vi "freq file -- file select controller.vi"(6 "Sweep folder path":path=path "\\\\rus-one\\newdata/data/Ultrasound/Experiment/ProbeTest/Probe10/Hg1201-4-C199-80K-1/Sweep1", 7 "action":T3=enum."init", 8 "Numeric":dbl, 11 "file select ref":refnum<vi>) -> (0 "file select OUT":T1={"from file "="1827_a", "load"=FALSE, "read from file list"=0, "folder kind"=enum."9w"} {"read from file list" items=["769_a", "841_a", "1399_a", "1502_a", "1527_a", "1705_a", "1916_a", "1958_a", "2061_a", "2227_a", "2365_a", "2551_a", "2713_a", "2761_a", "2964_a", "3000_a", "3030_a", "3084_a", "3235_a", "3366_a"]}, 1 "Numeric out":dbl, 3 "file select ref out":refnum<vi>)   [LabVIEW 2015]
uses:
  save-read action.ctl
  freq file -- file select control.ctl
  freq file -- file select folder control.ctl
  D:/github/resonant_ultrasound/maglab ultrasound -- arkady/file -- 9w path.vi
  D:/github/resonant_ultrasound/maglab ultrasound -- arkady/file -- open-create folder.vi
  <vilib>/regexp/Match Regular Expression.xnode
panel:
  in  "folder kind":T2=enum."9w"
  in  "file select":T1={"from file "="1827_a", "load"=FALSE, "read from file list"=0, "folder kind"=enum."9w"} {"read from file list" items=["769_a", "841_a", "1399_a", "1502_a", "1527_a", "1705_a", "1916_a", "1958_a", "2061_a", "2227_a", "2365_a", "2551_a", "2713_a", "2761_a", "2964_a", "3000_a", "3030_a", "3084_a", "3235_a", "3366_a"]}
  in  "load":bool caption="read"
  in  "regexp":string="(from file).*"
  in  "read from file list":u16(ring) items=["769_a", "841_a", "1399_a", "1502_a", "1527_a", "1705_a", "1916_a", "1958_a", "2061_a", "2227_a", "2365_a", "2551_a", "2713_a", "2761_a", "2964_a", "3000_a", "3030_a", "3084_a", "3235_a", "3366_a"]
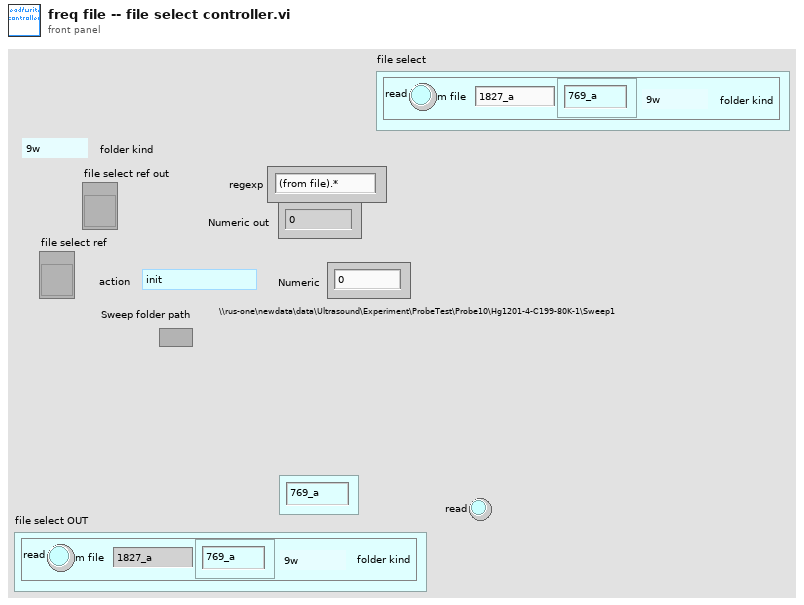
[diagram p1: front panel]
types:
  T1 = typedef "freq file -- file select control.ctl" = cluster{"from file ":string, "load":bool, "read from file list":u16, "folder kind":T2}
  T2 = typedef "freq file -- file select folder control.ctl" = enum16{"monitor", "9w"}
  T3 = typedef "save-read action.ctl" = enum16{"update save list", "update read list", "init", "check", "lookup read number", "lookup write number", "copy read from read ring", "saved file dirty", "saved file clean", "read file OK", "read file not OK", "nearest right", "nearest left", "increment read from", "copy read to save", "init save file", "erase event", "save event", "read event", "set save file", "decrement read from"}
  T4 = typedef "slide control.ctl" = cluster{"in slide":bool, "direction":bool, "start ":bool, "stop":bool, "next":bool}
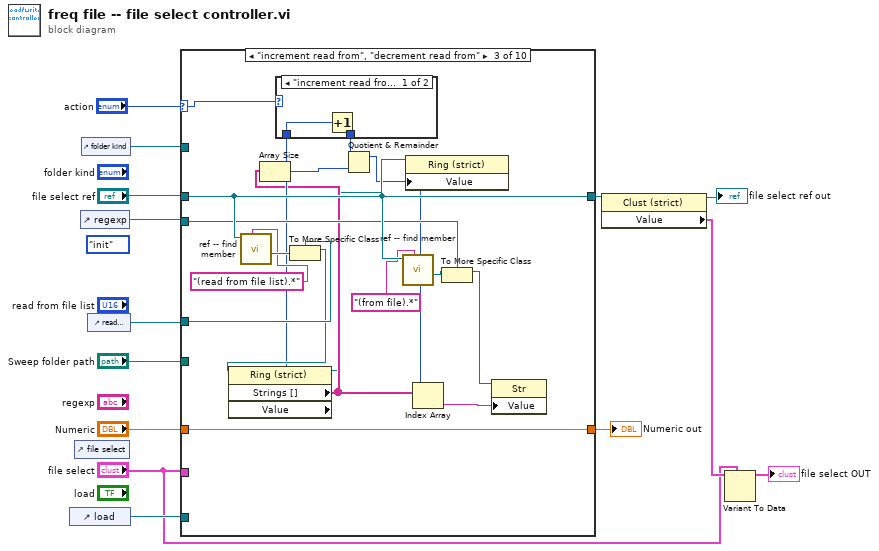
[diagram p0: block diagram]
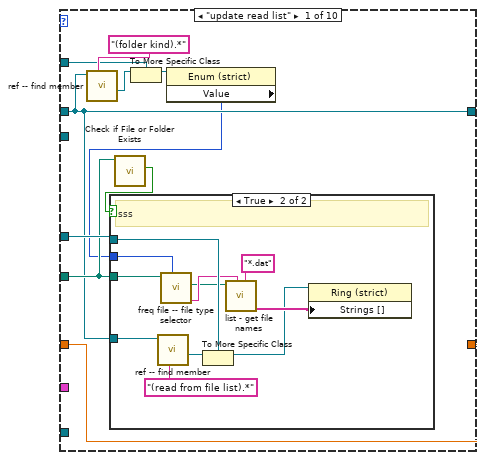
[diagram p2: hidden frame]
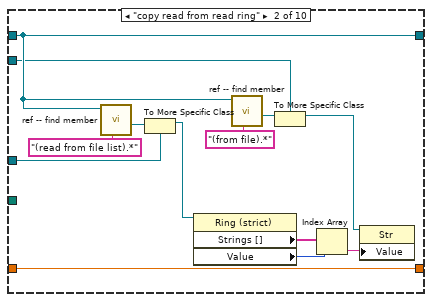
[diagram p4: hidden frame]
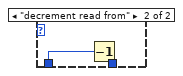
[diagram p5: hidden frame]
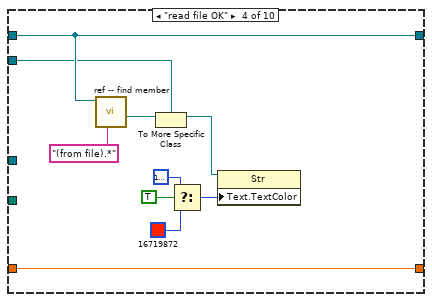
[diagram p6: hidden frame]
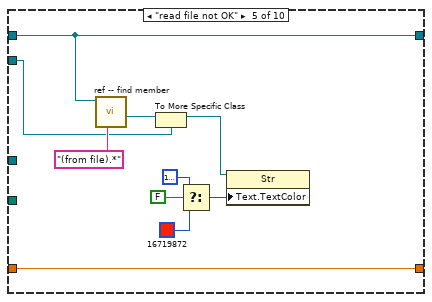
[diagram p7: hidden frame]
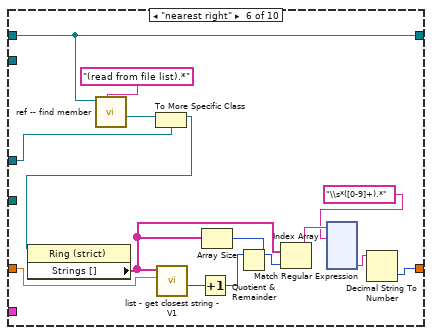
[diagram p8: hidden frame]
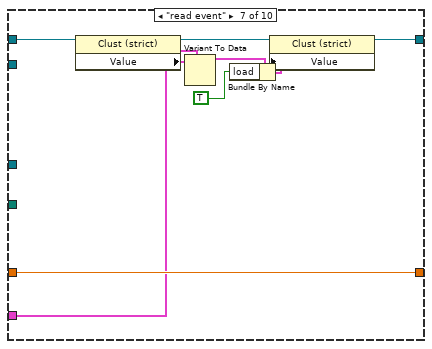
[diagram p9: hidden frame]
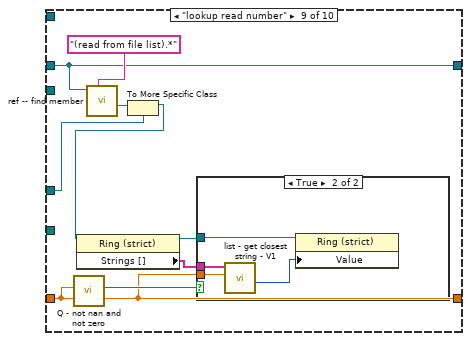
[diagram p11: hidden frame]
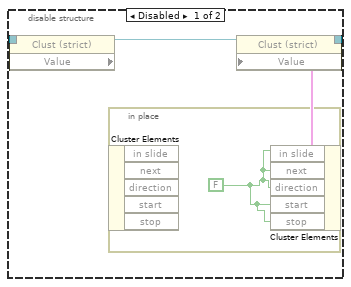
[diagram p14: hidden frame]
diagram:
  (unwired) save-read_action."init" ("action")
  n1 = control-ref of="load"() -> (w7:refnum<vi>)
  n2 = control-ref of="file select"() -> ()  [unwired: 1 out]
  n3 = control-ref of="regexp"() -> (w9:refnum<vi>)
  n4 = control-ref of="folder kind"() -> (w6:refnum<vi>)
  n5 = control-ref of="read from file list"() -> (w12:refnum<vi>)
  n6 = case shown="\"increment read from\", \"decrement read from\"" "action" {
    selector: "action" -> [_ _ w49 _ _ _ _ _ _ _]
    tunnel: "file select ref" -> [w19 w41 w61 w80 w90 w105 w225 w229 w232 w245]
    tunnel: [w19 w41 w61 w80 w90 w105 w222 w229 w232 w244] -> w2
    tunnel: "file select" -> [_ _ _ _ _ _ w224 _ _ _]
    tunnel: w12 -> [w24 w43 w63 _ _ w92 _ _ w235 _]
    tunnel: "Sweep folder path" -> [w23 _ _ _ _ _ _ _ _ _]
    tunnel: "Numeric" -> [w21 w36 w56 w71 w81 w91 w227 w228 w230 w243]
    tunnel: w9 -> [_ w39 w59 w78 w88 _ _ _ _ _]
    tunnel: [w21 w36 w56 w71 w81 w95 w227 w228 w230 w243] -> w8
    tunnel: w7 -> [_ _ _ _ _ _ _ _ _ _]
    tunnel: w6 -> [w17 _ _ _ _ _ _ _ _ _]
    frame "update read list" {
      n7 = call "ref -- find member.vi"("regexp"="(folder kind).*", "save/read ref"=w19) -> ("element"=w18:refnum<vi>)  [unwired: 7 in, 2 out]
      n8 = call <vilib>:"Check if File or Folder Exists.vi"("path"=w23) -> ("file or folder exists?"=w22:bool)  [unwired: 8 in, 2 out]
      n9 = To More Specific Class(target class=w17, reference=w18) -> (specific class reference=w16:refnum<vi>)  [unwired: 1 in, 1 out]
      n10 = property class="Enum (strict)"(reference=w16) -> ("Value"=w15:T2)  [unwired: 1 in, 2 out]
      n11 = case shown="True" w22 {
        tunnel: w24 -> [_ w33]
        tunnel: w19 -> [_ w31]
        tunnel: w23 -> [_ w28]
        tunnel: w15 -> [_ w25]
        frame False {
        }
        frame True {
          # "sss"
          n12 = call "ref -- find member.vi"("regexp"="(read from file list).*", "save/read ref"=w31) -> ("element"=w29:refnum<vi>)  [unwired: 7 in, 2 out]
          n13 = call "freq file -- file type selector.vi"("folder kind"=w25, "Sweep folder path"=w28) -> ("file name regular expression"=w27:string, "folder path"=w26:path)  [unwired: 7 in, 1 out]
          n14 = To More Specific Class(target class=w33, reference=w29) -> (specific class reference=w32:refnum<vi>)  [unwired: 1 in, 1 out]
          n15 = call "list - get file names.vi"("extension filter"="*.dat" ("pattern"), "regular expression"=w27, "folder path"=w26) -> ("Array"=w34:string[])  [unwired: 7 in, 1 out]
          n16 = property class="Ring (strict)"(reference=w32, "Strings []"=w34) -> ()  [unwired: 1 in, 2 out]
        }
      }
    }
    frame "copy read from read ring" {
      n17 = call "ref -- find member.vi"("regexp"="(read from file list).*", "save/read ref"=w41) -> ("element"=w45:refnum<vi>)  [unwired: 7 in, 2 out]
      n18 = To More Specific Class(target class=w43, reference=w45) -> (specific class reference=w42:refnum<vi>)  [unwired: 1 in, 1 out]
      n19 = property on="Property Node" class="Ring (strict)"(reference=w42) -> ("Strings []"=w48:string[], "Value"=w47:u16)  [unwired: 1 in, 2 out]
      n20 = call "ref -- find member.vi"("regexp"="(from file).*", "save/read ref"=w41) -> ("element"=w38:refnum<vi>)  [unwired: 7 in, 2 out]
      n21 = To More Specific Class(target class=w39, reference=w38) -> (specific class reference=w37:refnum<vi>)  [unwired: 1 in, 1 out]
      n22 = Index Array(array=w48, index=w47) -> (element=w46:string)
      n23 = property on="Property Node" class="Str"(reference=w37, "Value"=w46) -> ()  [unwired: 1 in, 2 out]
    }
    frame "increment read from", "decrement read from" {
      n24 = call "ref -- find member.vi"("regexp"="(read from file list).*", "save/read ref"=w61) -> ("element"=w65:refnum<vi>)  [unwired: 7 in, 2 out]
      n25 = To More Specific Class(target class=w63, reference=w65) -> (specific class reference=w62:refnum<vi>)  [unwired: 1 in, 1 out]
      n26 = property on="Property Node" class="Ring (strict)"(reference=w62) -> (reference out=w51:refnum<vi>, "Strings []"=w54:string[], "Value"=w55:u16)  [unwired: 1 in, 1 out]
      n27 = Array Size(array=w54) -> (size(s)=w53:i32)
      n28 = case shown="\"increment read from\", Default" w49 {
        tunnel: w55 -> [w68 w70]
        tunnel: [w67 w69] -> w52
        frame "increment read from", Default {
          n29 = Increment(x=w68) -> (x+1=w67:u16)
        }
        frame "decrement read from" {
          n30 = Decrement(x=w70) -> (x-1=w69:u16)
        }
      }
      n31 = Quotient & Remainder(x=w52, y=w53) -> (x-y*floor(x/y)=w50:i32)  [unwired: 1 out]
      n32 = call "ref -- find member.vi"("regexp"="(from file).*", "save/read ref"=w61) -> ("element"=w58:refnum<vi>)  [unwired: 7 in, 2 out]
      n33 = property on="Property Node" class="Ring (strict)"(reference=w51, "Value"=w50) -> ()  [unwired: 1 in, 2 out]
      n34 = Index Array(array=w54, index=w50) -> (element=w66:string)
      n35 = To More Specific Class(target class=w59, reference=w58) -> (specific class reference=w57:refnum<vi>)  [unwired: 1 in, 1 out]
      n36 = property on="Property Node" class="Str"(reference=w57, "Value"=w66) -> ()  [unwired: 1 in, 2 out]
    }
    frame "read file OK" {
      n37 = call "ref -- find member.vi"("regexp"="(from file).*", "save/read ref"=w80) -> ("element"=w77:refnum<vi>)  [unwired: 7 in, 2 out]
      n38 = To More Specific Class(target class=w78, reference=w77) -> (specific class reference=w73:refnum<vi>)  [unwired: 1 in, 1 out]
      n39 = Select(t=u32 16777222, s=TRUE, f=u32 16719872) -> (s? t:f=w74:u32)
      n40 = property on="Property Node" class="Str"(reference=w73, "Text.TextColor"=w74) -> ()  [unwired: 1 in, 2 out]
    }
    frame "read file not OK" {
      n41 = call "ref -- find member.vi"("regexp"="(from file).*", "save/read ref"=w90) -> ("element"=w87:refnum<vi>)  [unwired: 7 in, 2 out]
      n42 = To More Specific Class(target class=w88, reference=w87) -> (specific class reference=w83:refnum<vi>)  [unwired: 1 in, 1 out]
      n43 = Select(t=u32 16777222, s=FALSE, f=u32 16719872) -> (s? t:f=w84:u32)
      n44 = property on="Property Node" class="Str"(reference=w83, "Text.TextColor"=w84) -> ()  [unwired: 1 in, 2 out]
    }
    frame "nearest right" {
      n45 = call "ref -- find member.vi"("regexp"="(read from file list).*", "save/read ref"=w105) -> ("element"=w104:refnum<vi>)  [unwired: 7 in, 2 out]
      n46 = To More Specific Class(target class=w92, reference=w104) -> (specific class reference=w93:refnum<vi>)  [unwired: 1 in, 1 out]
      n47 = property class="Ring (strict)"(reference=w93) -> ("Strings []"=w99:string[])  [unwired: 1 in, 2 out]
      n48 = call "list - get closest string - V1.vi"("number"=w91, "string Array"=w99) -> ("closest index"=w103:i32)  [unwired: 7 in, 2 out]
      n49 = Increment(x=w103) -> (x+1=w102:i32)
      n50 = Array Size(array=w99) -> (size(s)=w101:i32)
      n51 = Quotient & Remainder(x=w102, y=w101) -> (x-y*floor(x/y)=w100:i32)  [unwired: 1 out]
      n52 = Index Array(array=w99, index=w100) -> (element=w98:string)
      n53 = xnode "Match Regular Expression"("input string"=w98, "regular expression"="\\s*([0-9]+).*") -> ("submatch 1"=w97:string)  [unwired: 4 in, 5 out]
      n54 = Decimal String To Number(string=w97) -> (number=w95:i32)  [unwired: 2 in, 1 out]
    }
    frame "read event" {
      n55 = property class="Clust (strict)"(reference=w225) -> (reference out=w223:refnum<vi>, "Value"=w226:T1)  [unwired: 1 in, 1 out]
      n56 = Variant To Data(type=w224, Variant=w226) -> (data=w221:T1)  [unwired: 1 in, 1 out]
      n57 = Bundle By Name(cluster=w221, "load"=TRUE ("Value")) -> (w220:T1)
      n58 = property class="Clust (strict)"(reference=w223, "Value"=w220) -> (reference out=w222:refnum<vi>)  [unwired: 1 in, 1 out]
    }
    frame "check", Default {
    }
    frame "lookup read number" {
      n59 = call "Q - not nan and not zero.vi"("Numeric"=w230) -> ("Boolean"=w238:bool)  [unwired: 10 in]
      n60 = call "ref -- find member.vi"("regexp"="(read from file list).*", "save/read ref"=w232) -> ("element"=w236:refnum<vi>)  [unwired: 7 in, 2 out]
      n61 = To More Specific Class(target class=w235, reference=w236) -> (specific class reference=w234:refnum<vi>)  [unwired: 1 in, 1 out]
      n62 = property class="Ring (strict)"(reference=w234) -> (reference out=w231:refnum<vi>, "Strings []"=w233:string[])  [unwired: 1 in, 1 out]
      n63 = case shown="True" w238 {
        tunnel: w233 -> [_ w242]
        tunnel: w230 -> [_ w241]
        tunnel: w231 -> [_ w240]
        frame False {
        }
        frame True {
          n64 = call "list - get closest string - V1.vi"("number"=w241, "string Array"=w242) -> ("closest index"=w239:i32)  [unwired: 7 in, 2 out]
          n65 = property class="Ring (strict)"(reference=w240, "Value"=w239) -> ()  [unwired: 1 in, 2 out]
        }
      }
    }
    frame "init" {
      n66 = disable-structure shown="Enabled" {
        disable-tunnel: w245 -> [w250 w252]
        disable-tunnel: [w248 w252] -> w244
        frame Disabled {
          n67 = property class="Clust (strict)"(reference=w250) -> (reference out=w249:refnum<vi>, "Value"=w246:T1)  [unwired: 1 in, 1 out]
          n68 = in-place {
            w251 = FALSE ("Boolean")
            n69 = in-place-cluster #1() -> ()  [unwired: 1 in, 5 out]
            n70 = in-place-cluster #1("in slide"=w251, "next"=w251, "direction"=w251, "start"=w251, "stop"=w251) -> (w247:T4)
          }
          n71 = property class="Clust (strict)"(reference=w249, "Value"=w247) -> (reference out=w248:refnum<vi>)  [unwired: 1 in, 1 out]
        }
        frame Enabled {
        }
      }
    }
  }
  "Numeric out" <- w8
  n72 = property class="Clust (strict)"(reference=w2) -> (reference out=→"file select ref out":refnum<vi>, "Value"=w13:T1)  [unwired: 1 in, 1 out]
  n73 = Variant To Data(type="file select", Variant=w13) -> (data=→"file select OUT":T1)  [unwired: 1 in, 1 out]
